vi "CMD_PARAM_SEND.vi"(0 "Input_Data":string[](array[string]), 5 "Error In":errorcluster) -> (12 "Validate CheckSum":bool, 13 "Command":u8[](array[numeric])=[5, 247, 4, 128, 255, 0, 0, 0, 0, 0, 0, 0, 0, 0] format="%x", 14 "Response":bool, 15 "Ack":bool, 16 "Command":bool, 17 "Add CheckSum":bool, 18 "Status":bool, 19 "Error Out":errorcluster)   [LabVIEW 2014]
panel:
  # "Flags"
  # "Param Send Command:"
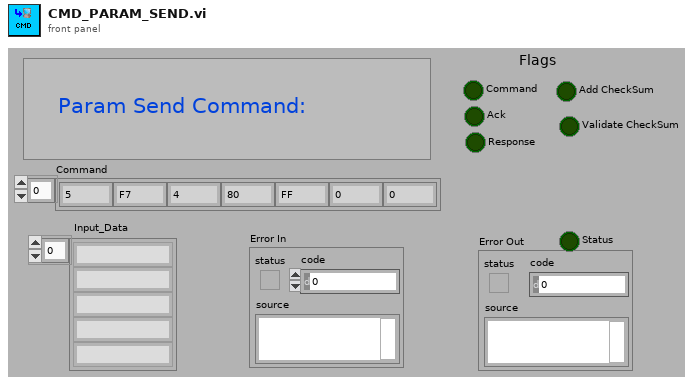
[diagram p1: front panel]
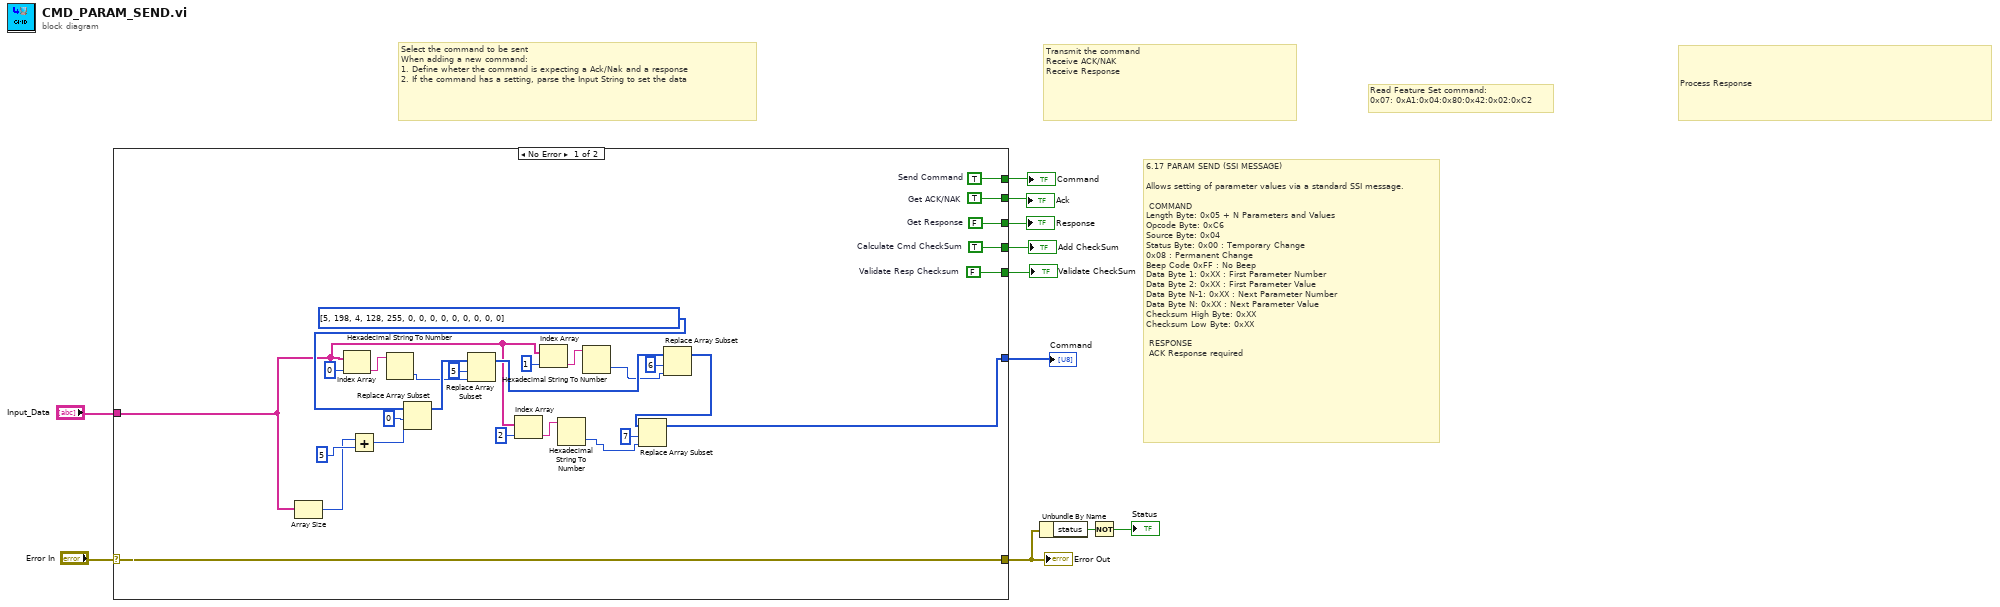
[diagram p0: block diagram]
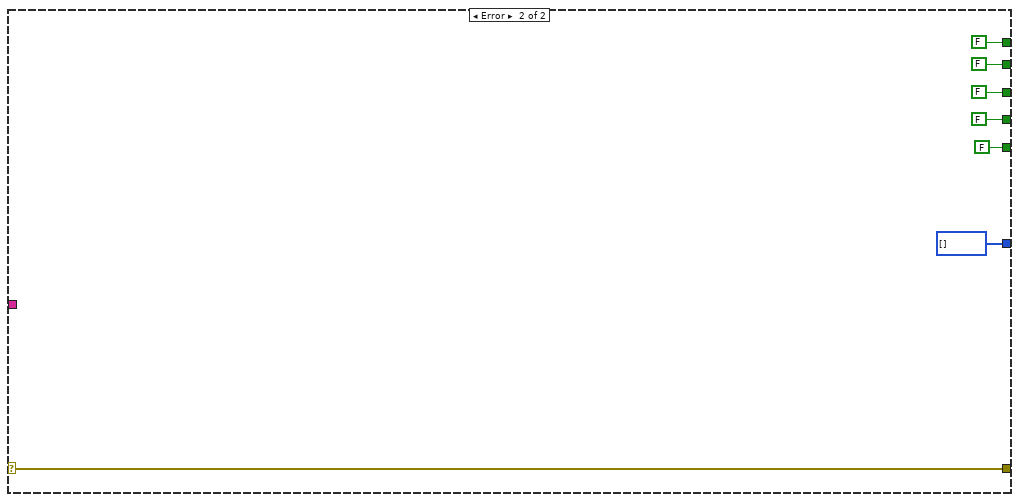
[diagram p2: hidden frame]
diagram:
  # "6.17\tPARAM SEND (SSI MESSAGE)\n\nAllows setting of parameter values via a standard SSI message.\n\n\tCOMMAND\nLength Byte:\t0x05 + N Parameters and Values\nOpcode Byte:\t0xC6\nSource Byte:\t0x04\nStatus Byte:\t0x00 : Temporary Change\n0x08 : Permanent Change\nBeep Code\t0xFF : No Beep\nData Byte 1:\t0xXX : First Parameter Number\nData Byte 2:\t0xXX : First Parameter Value\nData Byte N-1:\t0xXX : Next Parameter Number\nData Byte N:\t0xXX : Next Parameter Value\nChecksum High Byte:\t0xXX\nChecksum Low Byte:\t0xXX\n\n\tRESPONSE\n\tACK Response required"
  # "Read Feature Set command:\n0x07: 0xA1:0x04:0x80:0x42:0x02:0xC2"
  # "Process Response"
  # "Transmit the command\nReceive ACK/NAK\nReceive Response"
  # "Select the command to be sent\nWhen adding a new command:\n1. Define wheter the command is expecting a Ack/Nak and a response\n2. If the command has a setting, parse the Input String to set the data"
  n1 = case shown="No Error" "Error In" {
    selector: "Error In" -> [w35 w41]
    tunnel: [w39 FALSE ("Send Command")] -> w10
    tunnel: [w38 FALSE ("Get ACK/NAK")] -> w9
    tunnel: [w37 FALSE ("Get Response")] -> w8
    tunnel: [w36 FALSE ("Add CheckSum")] -> w7
    tunnel: [w13 u8[] []] -> w6
    tunnel: [w35 w41] -> w4
    tunnel: "Input_Data" -> [w12 _]
    tunnel: [w34 FALSE ("Validate Resp Checksum")] -> w1
    frame No Error {
      w34 = FALSE  # Validate Resp Checksum
      w36 = TRUE  # Calculate Cmd CheckSum
      w37 = FALSE  # Get Response
      w39 = TRUE  # Send Command
      w38 = TRUE  # Get ACK/NAK
      n2 = Array Size(array=w12) -> (size(s)=w14:i32)
      n3 = Index Array(array=w12, index=0) -> (element=w33:string)
      n4 = Add(x=w14, y=5) -> (x+y=w18:i32)
      n5 = Hexadecimal String To Number(string=w33) -> (number=w17:u32)  [unwired: 2 in, 1 out]
      n6 = Replace Array Subset(array=u8[] [5, 198, 4, 128, 255, 0, 0, 0, 0, 0, 0, 0, 0, 0], new element=w18, index=0) -> (w28:u8[])
      n7 = Replace Array Subset(array=w28, new element=w17, index=5) -> (w24:u8[])
      n8 = Index Array(array=w12, index=2) -> (element=w23:string)
      n9 = Index Array(array=w12, index=1) -> (element=w27:string)
      n10 = Hexadecimal String To Number(string=w23) -> (number=w15:u32)  [unwired: 2 in, 1 out]
      n11 = Hexadecimal String To Number(string=w27) -> (number=w16:u32)  [unwired: 2 in, 1 out]
      n12 = Replace Array Subset(array=w24, new element=w16, index=6) -> (w20:u8[])
      n13 = Replace Array Subset(array=w20, new element=w15, index=7) -> (w13:u8[])
    }
    frame Error {
    }
  }
  "Error Out" <- w4
  "Command" <- w10
  "Ack" <- w9
  "Response" <- w8
  "Add CheckSum" <- w7
  "Command" <- w6
  "Validate CheckSum" <- w1
  n14 = Unbundle By Name(w4) -> ("status"=w3:bool)
  n15 = Not(x=w3) -> (.not. x?=→"Status":bool)
